vi "Write Pressure Transducer Compensator.vi"(10 "Pressure Transducer Compensator":T1={"PID Gains"={"Proportional Gain (Kc)"=1.0, "Integral Time (Ti, min)"=0.01, "Derivative Time (Td, min)"=0.0}, "Pressure Transducer Output Range"={"High"=0.0, "Low"=0.0}, "Vcoil"=1.0} {"Pressure Transducer Output Range"."Low" min=-888.0 max=888.0 format="%.2f"; "Pressure Transducer Output Range"."High" min=-888.0 max=888.0 format="%.2f"; "Vcoil" format="%.3f"; "PID Gains"."Derivative Time (Td, min)" format="%.3f"; "PID Gains"."Integral Time (Ti, min)" format="%.3f"; "PID Gains"."Proportional Gain (Kc)" format="%.3f"}, 11 "PressureTransducerCompensator in":refnum<class "PressureTransducerCompensator.lvclass">) -> (3 "PressureTransducerCompensator out":refnum<class "PressureTransducerCompensator.lvclass">)   [LabVIEW 2013, in "PressureTransducerCompensator.lvclass"]
uses:
  PressureTransducerCompensator.lvclass
  Configuration/PressureTransducerCompensator.ctl
  Configuration/PIDGains.ctl
  Configuration/PressureTransducerOutputRange.ctl
  PressureTransducerCompensator.lvclass/PressureTransducerCompensator.ctl
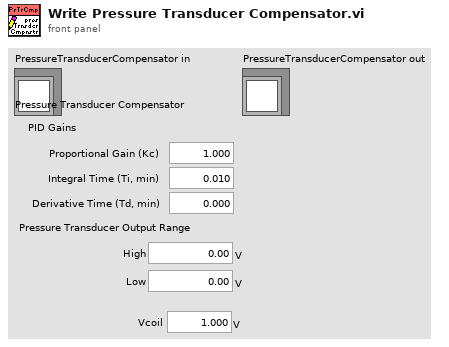
[diagram p1: front panel]
types:
  T1 = typedef "PressureTransducerCompensator.ctl" = cluster{"PID Gains":T2, "Pressure Transducer Output Range":T3, "Vcoil":dbl[unit]}
  T2 = typedef "PIDGains.ctl" = cluster{"Proportional Gain (Kc)":dbl, "Integral Time (Ti, min)":dbl, "Derivative Time (Td, min)":dbl}
  T3 = typedef "PressureTransducerOutputRange.ctl" = cluster{"High":dbl[unit], "Low":dbl[unit]}
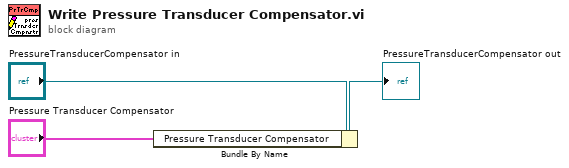
[diagram p0: block diagram]
diagram:
  n1 = Bundle By Name(cluster="PressureTransducerCompensator in", "Pressure Transducer Compensator"="Pressure Transducer Compensator") -> (→"PressureTransducerCompensator out":refnum<class "PressureTransducerCompensator.lvclass">)
